vi "Read Typedef Description.vi"   [LabVIEW 2019, in "JSON-Schema.lvlib"]
uses:
  JSON-Schema.lvlib
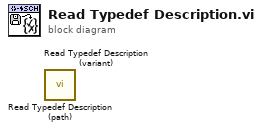
[diagram p0: block diagram]
diagram:
  n1 = call "Read Typedef Description (path).vi"() -> ()  [unwired: 9 in, 3 out]
  n2 = call "Read Typedef Description (variant).vi"() -> ()  [unwired: 9 in, 3 out]
